vi "main_program.vi"() -> ()   [LabVIEW 2016]
panel:
  in  "file path (use dialog)":path
  in  "total g-code line":i32
  out "N instruction":i32
  out "servo initial":dbl
  out "y initial":dbl
  out "x initial":dbl
  out "speed (ms)":dbl
  out "delay (ms)":dbl
  out "servo angle":dbl
  out "currently instruction":string
  # "This program is interpreted the g-code file."
  # "PLEASE enter the total number of g-code line and path of g-code."
  # "DISPLAY"
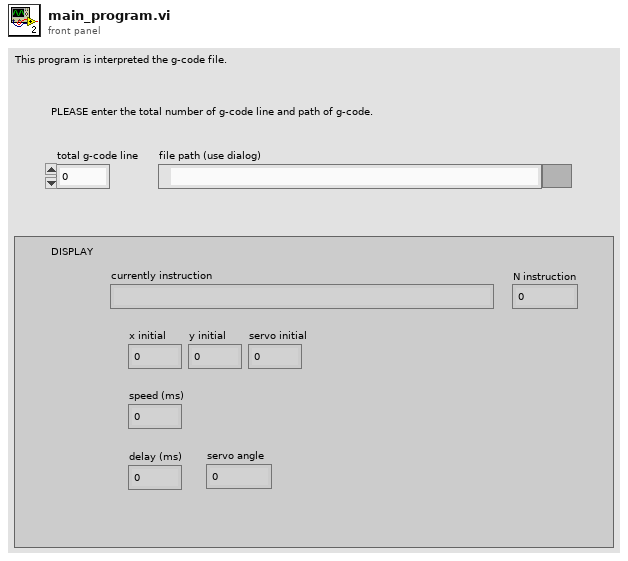
[diagram p1: front panel]
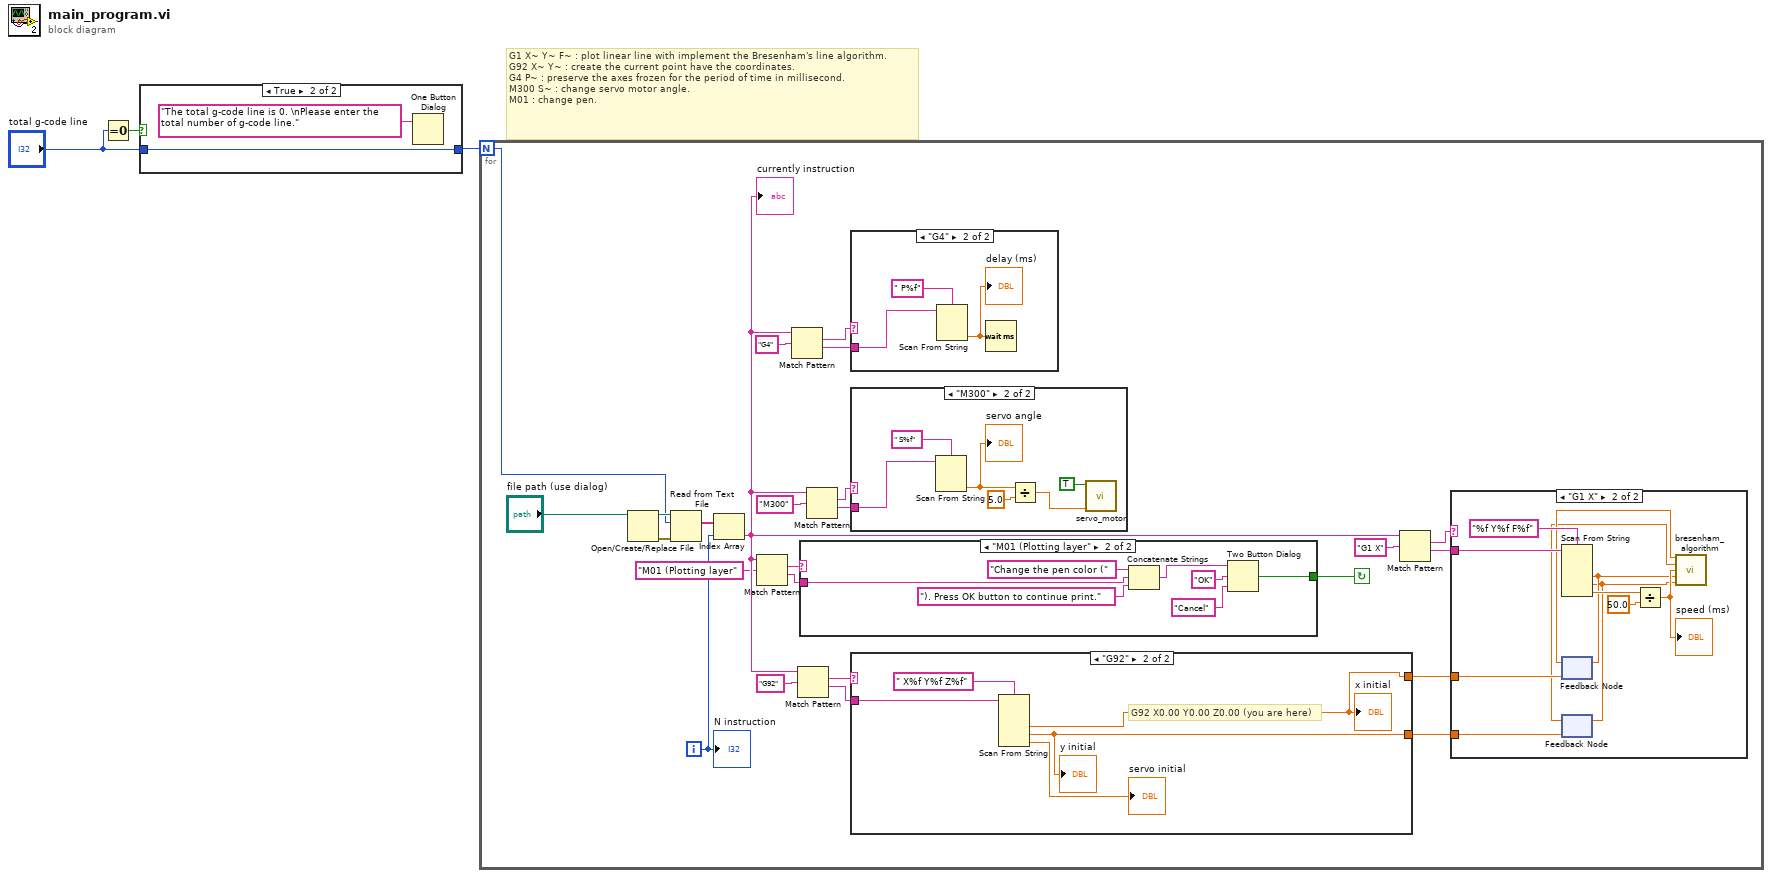
[diagram p0: block diagram]
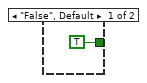
[diagram p3: hidden frame]
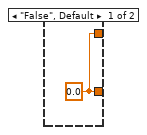
[diagram p4: hidden frame]
diagram:
  # "G1 X~ Y~ F~ : plot linear line with implement the Bresenham's line algorithm.\nG92 X~ Y~ : create the current point have the coordinates.\nG4 P~ : preserve the axes frozen for the period of time in millisecond. \nM300 S~ : change servo motor angle. \nM01 : change pen."
  n1 = Equal To 0?(x="total g-code line") -> (x = 0?=w3:bool)
  n2 = case shown="True" w3 {
    tunnel: "total g-code line" -> [w4 w5]
    tunnel: [w4 w5] -> w1
    frame False {
    }
    frame True {
      n3 = One Button Dialog(message="The total g-code line is 0. \nPlease enter the total number of g-code line.") -> ()  [unwired: 1 in, 1 out]
    }
  }
  n4 = for {
    N: w1 -> [w28]
    i -> [w27]
    stop <- w7 continue-if-true
    n5 = Open/Create/Replace File(file path (use dialog)="file path (use dialog)") -> (refnum out=w30:refnum<file>, error out=w29:errorcluster)  [unwired: 5 in, 1 out]
    n6 = Read from Text File(file (use dialog)=w30, count=w28, error in=w29) -> (text=w26:string[])  [unwired: 1 in, 3 out]
    n7 = Index Array(array=w26, index=w27) -> (element=w11:string)
    "currently instruction" <- w11
    n8 = Match Pattern(string=w11, regular expression="M01 (Plotting layer") -> (match substring=w9:string, after substring=w8:string)  [unwired: 1 in, 2 out]
    n9 = Match Pattern(string=w11, regular expression="G4") -> (match substring=w21:string, after substring=w20:string)  [unwired: 1 in, 2 out]
    n10 = Match Pattern(string=w11, regular expression="G92") -> (match substring=w16:string, after substring=w14:string)  [unwired: 1 in, 2 out]
    n11 = case shown="\"M01 (Plotting layer\"" w9 {
      tunnel: w8 -> [_ w38]
      tunnel: [TRUE w33] -> w7
      frame "False", Default {
      }
      frame "M01 (Plotting layer" {
        n12 = Concatenate Strings("Change the pen color (" ("string"), w38, "). Press OK button to continue print." ("string")) -> (w36:string)
        n13 = Two Button Dialog(message=w36, 1:"Cancel" ("F button name (\"Cancel\")"), 2:"OK" ("T button name (\"OK\")")) -> (T button?=w33:bool)
      }
    }
    n14 = Match Pattern(string=w11, regular expression="M300") -> (match substring=w23:string, after substring=w24:string)  [unwired: 1 in, 2 out]
    n15 = case shown="\"G4\"" w21 {
      tunnel: w20 -> [_ w59]
      frame "False", Default {
      }
      frame "G4" {
        n16 = Scan From String(format string=" P%f", input string=w59) -> (output 1=w57:dbl)  [unwired: 3 in, 3 out]
        "delay (ms)" <- w57
        n17 = Wait (ms)(milliseconds to wait=w57) -> ()  [unwired: 1 out]
      }
    }
    n18 = case shown="\"M300\"" w23 {
      tunnel: w24 -> [_ w64]
      frame "False", Default {
      }
      frame "M300" {
        n19 = Scan From String(format string=" S%f", input string=w64) -> (output 1=w61:dbl)  [unwired: 3 in, 3 out]
        "servo angle" <- w61
        n20 = Divide(x=w61, y=5.0) -> (x/y=w60:dbl)
        n21 = call "servo_motor.vi"("Duty Cycle"=w60, "Enable Outputs"=TRUE) -> ()  [unwired: 9 in, 1 out]
      }
    }
    n22 = case shown="\"G92\"" w16 {
      tunnel: w14 -> [_ w44]
      tunnel: [w40 w42] -> w13
      tunnel: [w40 w41] -> w12
      frame "False", Default {
        w40 = 0.0 ("x initial")
      }
      frame "G92" {
        # "G92 X0.00 Y0.00 Z0.00 (you are here)"
        n23 = Scan From String(format string=" X%f Y%f Z%f", input string=w44) -> (output 1=w42:dbl, output 2=w41:dbl, output 3=→"servo initial":dbl)  [unwired: 5 in, 3 out]
        "x initial" <- w42
        "y initial" <- w41
      }
    }
    n24 = Match Pattern(string=w11, regular expression="G1 X") -> (match substring=w18:string, after substring=w17:string)  [unwired: 1 in, 2 out]
    n25 = case shown="\"G1 X\"" w18 {
      tunnel: w17 -> [_ w55]
      tunnel: w13 -> [_ w51]
      tunnel: w12 -> [_ w49]
      frame "False", Default {
      }
      frame "G1 X" {
        n26 = Scan From String(format string="%f Y%f F%f", input string=w55) -> (output 1=w47:dbl, output 2=w46:dbl, output 3=w54:dbl)  [unwired: 5 in, 3 out]
        n27 = feedback-in #1(w47) -> ()
        n28 = feedback #1(w51) -> (w52:dbl)
        n29 = feedback #2(w49) -> (w50:dbl)
        n30 = feedback-in #2(w46) -> ()
        n31 = Divide(x=w54, y=50.0) -> (x/y=w48:dbl)
        "speed (ms)" <- w48
        n32 = call "bresenham_algorithm.vi"("pX"=w52, "pY"=w50, "speed (ms)"=w48, "newX"=w47, "newY"=w46) -> ()  [unwired: 11 in]
      }
    }
    "N instruction" <- w27
  }
